vi "Manlight - Update Power.vi"(4 "error in (no error)":errorcluster, 6 "VISA resource name":refnum<visa-resource-name>, 7 "params":variant) -> (0 "error out":errorcluster, 2 "VISA resource name out":refnum<visa-resource-name>)   [LabVIEW 2020]
uses:
  _Controls/Manlight Controls.ctl
panel:
  out "return count":u32
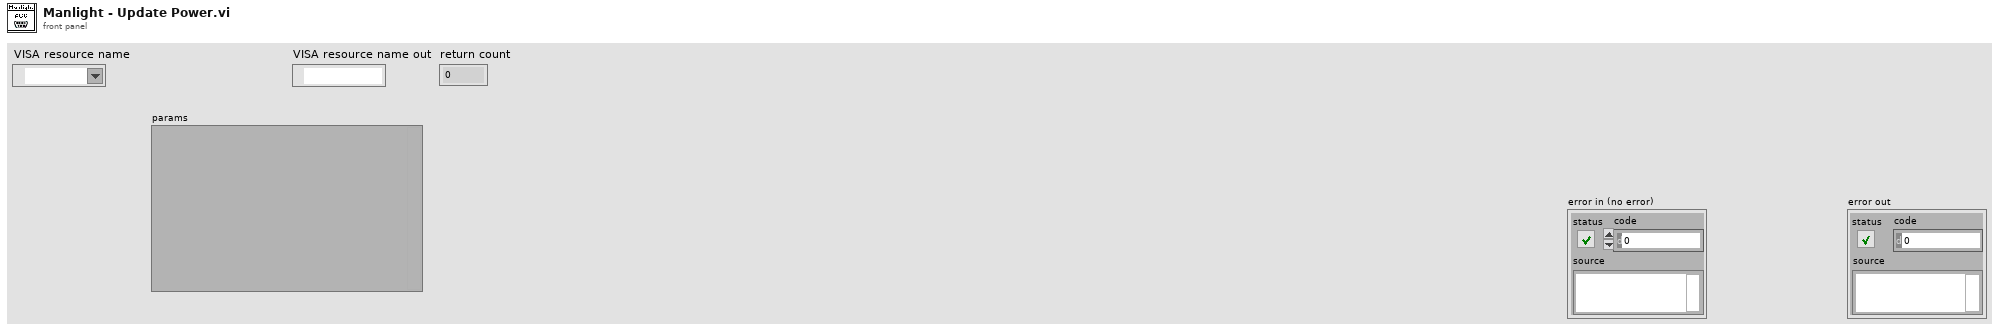
[diagram p1: front panel]
types:
  T1 = typedef "Manlight Controls.ctl" = cluster{"Manlight Power":dbl, "Open Serial":bool, "VISA Refnum":refnum<visa-resource-name>}
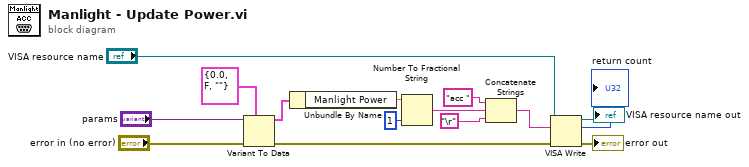
[diagram p0: block diagram]
diagram:
  n1 = Variant To Data(error in="error in (no error)", type=T1 {"Manlight Power"=0.0, "Open Serial"=FALSE, "VISA Refnum"=""} ("Manlight Controls"), Variant="params") -> (data=w5:T1, error out=w7:errorcluster)
  n2 = Unbundle By Name(w5) -> ("Manlight Power"=w4:dbl)
  n3 = Number To Fractional String(number=w4, precision (6)=i16 1) -> (F-format string=w12:string)  [unwired: 2 in]
  n4 = Concatenate Strings("acc ", w12, "\r") -> (w14:string)
  n5 = VISA Write(VISA resource name="VISA resource name", write buffer=w14, error in (no error)=w7) -> (VISA resource name out=→"VISA resource name out":refnum<visa-resource-name>, return count=→"return count":u32, error out=→"error out":errorcluster)
